vi "2photocell+ledcontrol+sum_cal2.vi"() -> ()   [LabVIEW 2016]
uses:
  <vilib>/LabVIEW Interface for Arduino/LabVIEW Interface for Arduino.lvlib
  <vilib>/ptbypt/NI_PtbyPt.lvlib
panel:
  in  "stop":bool
  in  "Tab Control":enum32{"Page 1", "Page 2", "Page 3"}(tab)
  out "Voltage":dbl(knob) scale=0.0..5.0
  out "Filtered x":dbl format="%0.2f"
  out "alarm":bool
  out "LUX":string="Error"
  in  "br_coef":dbl
  in  "thrs low":i32=1
  in  "thrs high":i32=4
  in  "q":dbl
  in  "p":dbl
  in  "k":dbl
  in  "thrs up":dbl
  in  "thrs down":dbl
  in  "Slide 3":dbl(slide) min=0.0 max=255.0 scale=0.0..255.0
  in  "Slide 2":dbl(slide) min=0.0 max=255.0 scale=0.0..255.0
  in  "Slide":dbl(slide) min=0.0 max=255.0 scale=0.0..255.0
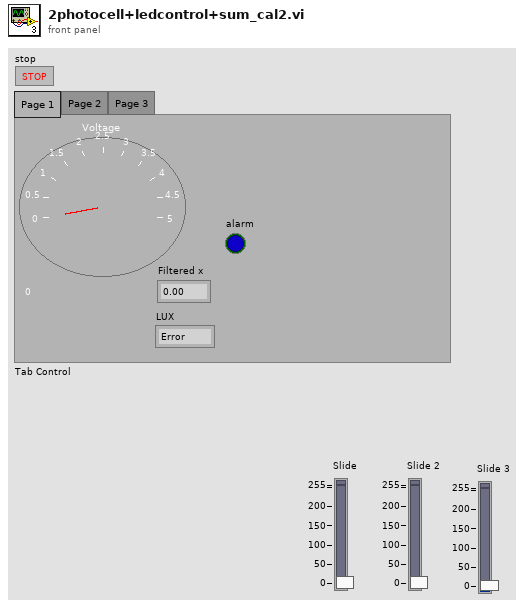
[diagram p1: front panel]
types:
  T1 = typedef "LabVIEW Interface for Arduino.lvlib/Arduino Resource.ctl" = cluster{"VISA resource":refnum<visa-resource-name>, "Board Type":T2, "Connection Type":enum8{"USB / Serial"}, "Bytes Per Packet (15)":u8}
  T2 = typedef "LabVIEW Interface for Arduino.lvlib/Board Type.ctl" = enum16{"Uno", "Dimuelanove w/Atmega 328", "Mega 2560"}
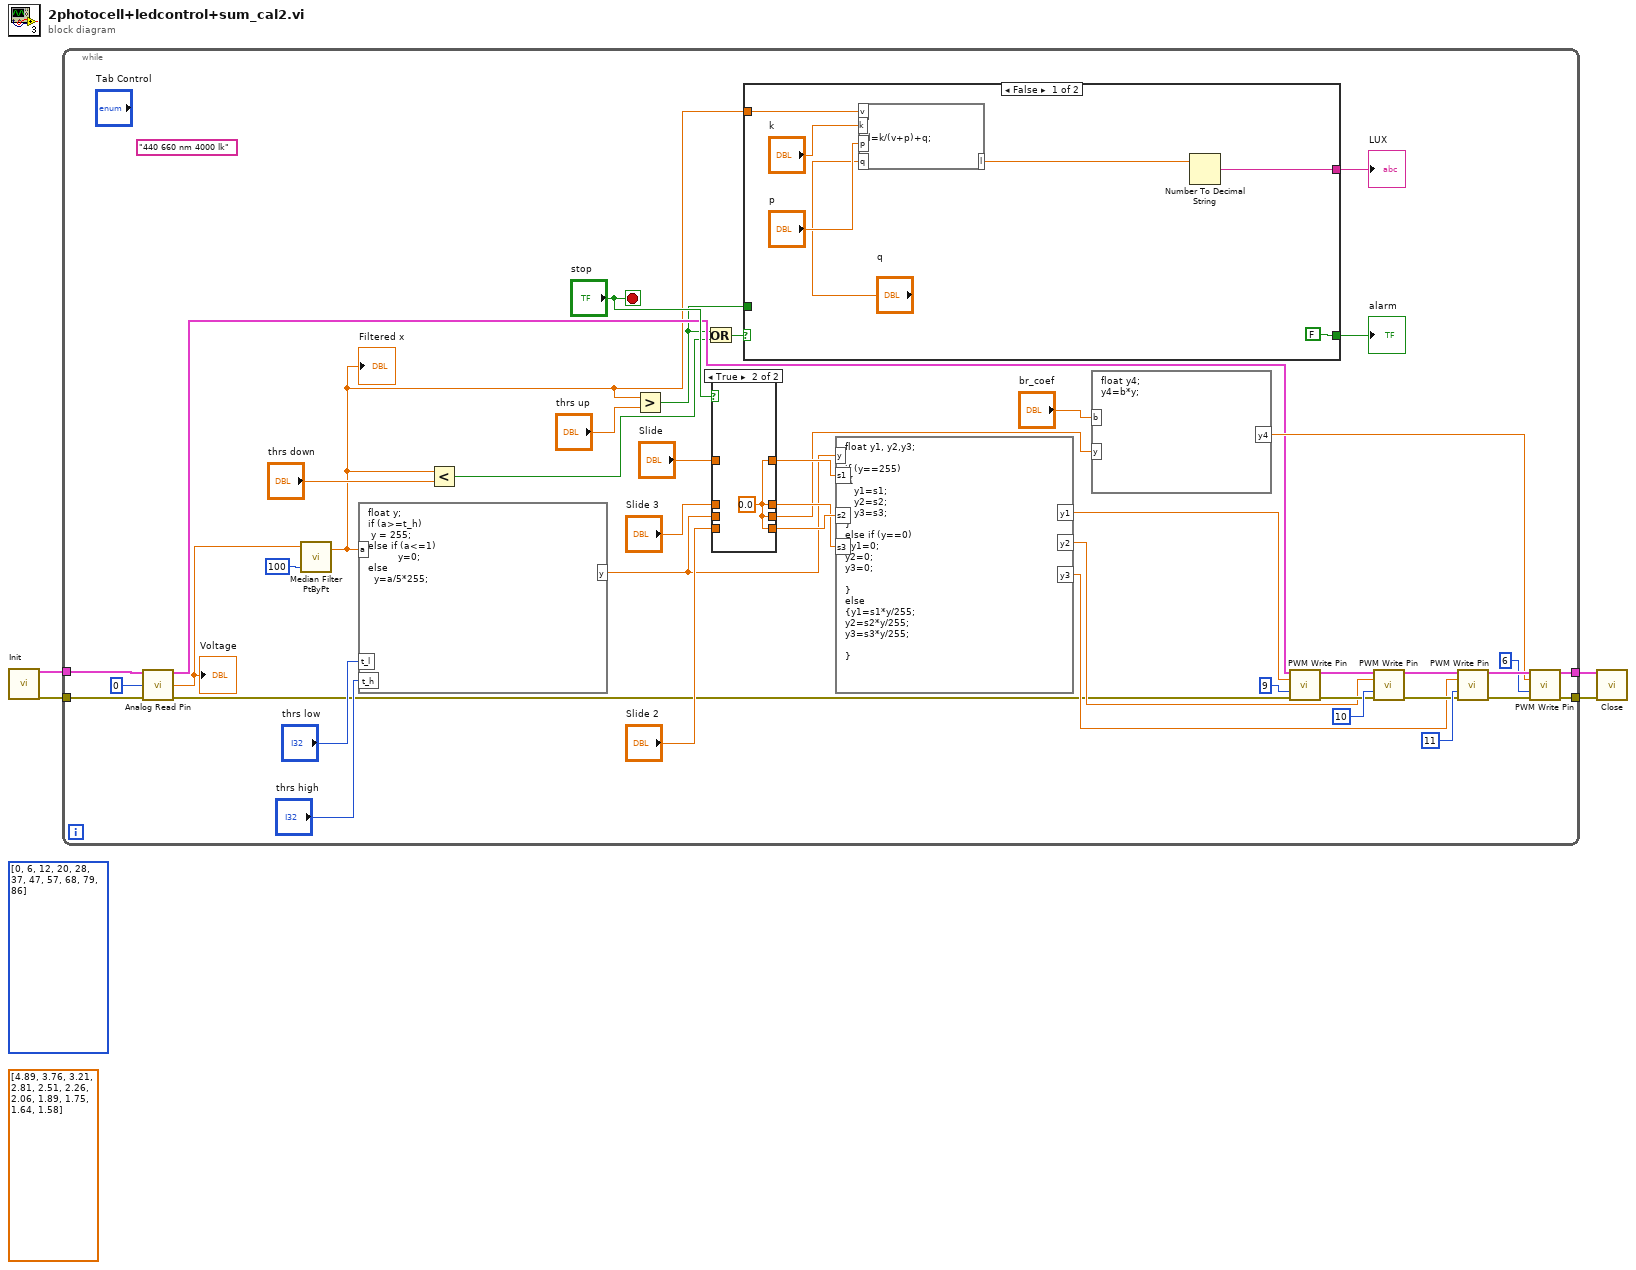
[diagram p0: block diagram]
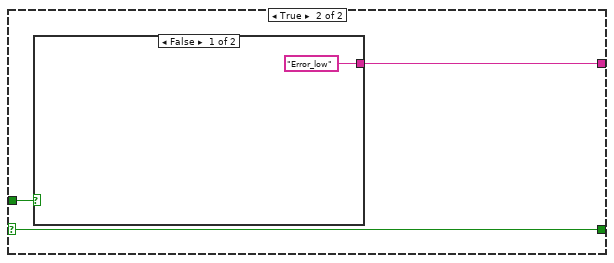
[diagram p2: hidden frame]
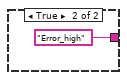
[diagram p3: hidden frame]
diagram:
  (unwired) dbl[] [4.89, 3.76, 3.21, 2.81, 2.51, 2.26, 2.06, 1.89, 1.75, 1.64, 1.58]
  (unwired) i32[] [0, 6, 12, 20, 28, 37, 47, 57, 68, 79, 86]
  n1 = call <vilib>:"Init.vi"() -> ("Arduino Resource"=w3:T1, "error out"=w4:errorcluster)  [unwired: 18 in]
  n2 = while {
    tunnel: w4 -> [w46]
    tunnel: w3 -> [w44]
    tunnel: [w22] -> w2
    tunnel: [w21] -> w1
    stop <- "stop" stop-if-true
    (unwired) "440 660 nm 4000 lk"
    n3 = call <vilib>:"Analog Read Pin.vi"("Arduino Resource"=w44, "Analog Input Pin (0)"=u8 0, "error in"=w46) -> ("Arduino Resource"=w14:T1, "Voltage"=w43:dbl, "error out"=w13:errorcluster)  [unwired: 10 in]
    "Voltage" <- w43
    n4 = call <vilib>:"Median Filter PtByPt.vi"("rank"=100, "x"=w43) -> ("Filtered x"=w7:dbl)  [unwired: 2 in, 1 out]
    "Filtered x" <- w7
    n5 = formula code="float y;\nif (a>=t_h)\n y = 255;\nelse if (a<=1)\n          y=0;\nelse\n  y=a/5*255;"("a"=w7, "t_l"="thrs low", "t_h"="thrs high") -> ("y"=w18:dbl)
    n6 = Less?(x=w7, y="thrs down") -> (x < y?=w10:bool)
    n7 = Greater?(x=w7, y="thrs up") -> (0:w5:bool)
    n8 = Or(x=w5, y=w10) -> (x .or. y?=w9:bool)
    n9 = case shown="True" "stop" {
      tunnel: "Slide 2" -> [w63 _]
      tunnel: [w63 w64] -> w28
      tunnel: "Slide 3" -> [w62 _]
      tunnel: [w62 w64] -> w27
      tunnel: "Slide" -> [w61 _]
      tunnel: [w61 w64] -> w29
      tunnel: w18 -> [w60 _]
      tunnel: [w60 w64] -> w16
      frame False {
      }
      frame True {
        w64 = 0.0 ("Slide 2")
      }
    }
    n10 = case shown="False" w9 {
      selector: w9 -> [_ w57]
      tunnel: [FALSE w57] -> w8
      tunnel: w7 -> [w53 _]
      tunnel: [w51 w55] -> w6
      tunnel: w5 -> [_ w56]
      frame False {
        n11 = formula code="l=k/(v+p)+q;"("v"=w53, "k"="k", "p"="p", "q"="q") -> ("l"=w52:dbl)
        n12 = Number To Decimal String(number=w52) -> (decimal integer string=w51:string)  [unwired: 1 in]
      }
      frame True {
        n13 = case shown="False" w56 {
          tunnel: ["Error_low" "Error_high"] -> w55
          frame False {
          }
          frame True {
          }
        }
      }
    }
    "alarm" <- w8
    "LUX" <- w6
    n14 = formula code="float y1, y2,y3;\n\nif (y==255)\n {\n   y1=s1;\n   y2=s2;\n   y3=s3;\n}\nelse if (y==0)\n{y1=0;\ny2=0;\ny3=0;\n\n}\nelse \n{y1=s1*y/255;\ny2=s2*y/255;\ny3=s3*y/255;\n\n}"("s1"=w29, "s2"=w28, "s3"=w27, "y"=w18) -> ("y1"=w26:dbl, "y2"=w25:dbl, "y3"=w24:dbl)
    n15 = formula code="float y4;\ny4=b*y;"("b"="br_coef", "y"=w16) -> ("y4"=w15:dbl)
    n16 = call <vilib>:"PWM Write Pin.vi"("Arduino Resource"=w14, "Duty Cycle (0 - 255)"=w26, "PWM Pin (3)"=u8 9, "error in"=w13) -> ("Arduino Resource"=w35:T1, "error out"=w31:errorcluster)  [unwired: 10 in]
    n17 = call <vilib>:"PWM Write Pin.vi"("Arduino Resource"=w35, "Duty Cycle (0 - 255)"=w25, "PWM Pin (3)"=u8 10, "error in"=w31) -> ("Arduino Resource"=w34:T1, "error out"=w30:errorcluster)  [unwired: 10 in]
    n18 = call <vilib>:"PWM Write Pin.vi"("Arduino Resource"=w34, "Duty Cycle (0 - 255)"=w24, "PWM Pin (3)"=u8 11, "error in"=w30) -> ("Arduino Resource"=w23:T1, "error out"=w20:errorcluster)  [unwired: 10 in]
    n19 = call <vilib>:"PWM Write Pin.vi"("Arduino Resource"=w23, "Duty Cycle (0 - 255)"=w15, "PWM Pin (3)"=u8 6, "error in"=w20) -> ("Arduino Resource"=w22:T1, "error out"=w21:errorcluster)  [unwired: 10 in]
  }
  n20 = call <vilib>:"Close.vi"("Arduino Resource"=w2, "error in"=w1) -> ()  [unwired: 13 in, 1 out]
